vi "UpdateGraph (SubVI).vi"(6 "x":dbl[](array[numeric]), 9 "Y2":dbl[](array[numeric]), 10 "Y1":dbl[](array[numeric]), 11 "XYGraph (Eingang)":refnum<vi>) -> ()   [LabVIEW 2014]
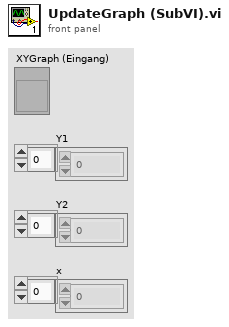
[diagram p1: front panel]
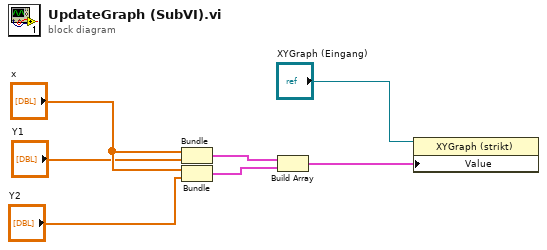
[diagram p0: block diagram]
diagram:
  n1 = Bundle("x"="x", "Y1"="Y1") -> (w3:cluster{"x":dbl[], "Y1":dbl[]})  [unwired: 1 in]
  n2 = Bundle("x"="x", "Y2"="Y2") -> (w4:cluster{"x":dbl[], "Y2":dbl[]})  [unwired: 1 in]
  n3 = Build Array(w3, w4) -> (w2:cluster{"x":dbl[], "Y2":dbl[]}[])
  n4 = property class="XYGraph (strikt)"(reference="XYGraph (Eingang)", "Value"=w2) -> ()  [unwired: 1 in, 2 out]
